vi "Driver Init.vi"(8 "error in (no error)":errorcluster, 11 "DriverMasterAsync in":refnum<class "DriverMasterAsync.lvclass">) -> (0 "error out":errorcluster, 3 "DriverMasterAsync out":refnum<class "DriverMasterAsync.lvclass">)   [LabVIEW 2014, in "DriverMasterAsync.lvlib" / "DriverMasterAsync.lvclass"]
uses:
  DriverMasterAsync.lvclass
  APIs/Data Queue/Async Acquisition Data Cluster.ctl
  DriverMasterAsync.lvclass/DriverMasterAsync.ctl
  APIs/Data Queue/WINFAS 2 Data Queue.lvlib
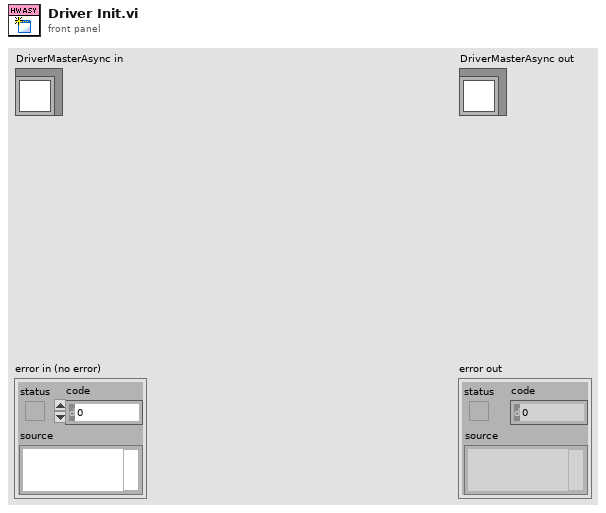
[diagram p1: front panel]
types:
  T1 = typedef "WINFAS 2 Data Queue.lvlib/Async Acquisition Data Cluster.ctl" = cluster{"Data":sgl[]}
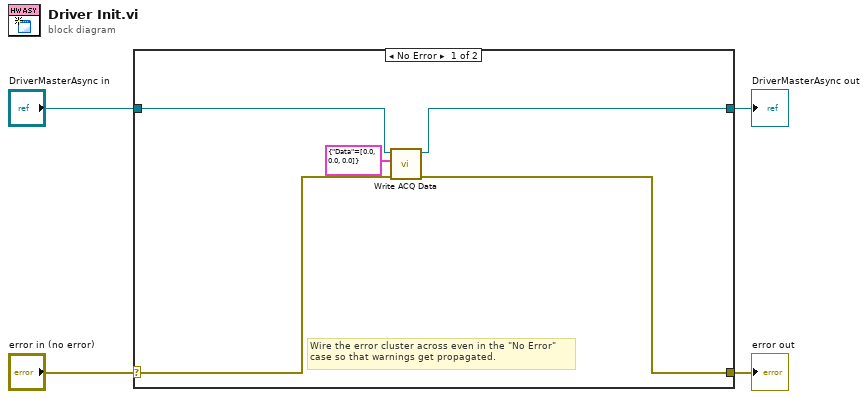
[diagram p0: block diagram]
diagram:
  n1 = case shown="No Error" "error in (no error)" {
    selector: "error in (no error)" -> [w7 w11]
    tunnel: [w6 w11] -> w3
    tunnel: [w8 w10] -> w1
    tunnel: "DriverMasterAsync in" -> [w9 w10]
    frame No Error {
      # "Wire the error cluster across even in the \"No Error\"\ncase so that warnings get propagated."
      n2 = call "Write ACQ Data.vi"("error in (no error)"=w7, "ACQ Data"=T1 {"Data"=[0.0, 0.0, 0.0]}, "DriverMasterAsync in"=w9) -> ("error out"=w6:errorcluster, "DriverMasterAsync out"=w8:refnum<class "DriverMasterAsync.lvclass">)  [unwired: 7 in]
    }
    frame Error {
    }
  }
  "error out" <- w3
  "DriverMasterAsync out" <- w1
